vi "NT Write Generic Value.vi"(8 "error in":errorcluster, 9 "Owning Write":bool, 10 "Field Value":T1, 11 "Name":string="Boolean") -> (0 "error out":errorcluster)   [LabVIEW 2017]
doc: "Write the generic cluster data for a variable into the named entry."
uses:
  <vilib>/Rock Robotics/Network Tables/Field Data.ctl
  <vilib>/Rock Robotics/Network Tables/Field Type.ctl
  <vilib>/Rock Robotics/Network Tables/Sequence.ctl
  <vilib>/Rock Robotics/Network Tables/Make Table Operation.ctl
  <vilib>/Rock Robotics/Network Tables/Manage Dirty Field ID List.vi
  <vilib>/Rock Robotics/Network Tables/NT Globals.vi
  <vilib>/Rock Robotics/Network Tables/Update Other Clients.vi
  <vilib>/Rock Robotics/Network Tables/Build Entry Assign Buffer.vi
  <vilib>/Rock Robotics/Network Tables/Field Data Manager.vi
  <vilib>/Rock Robotics/Network Tables/Usage Statistics.vi
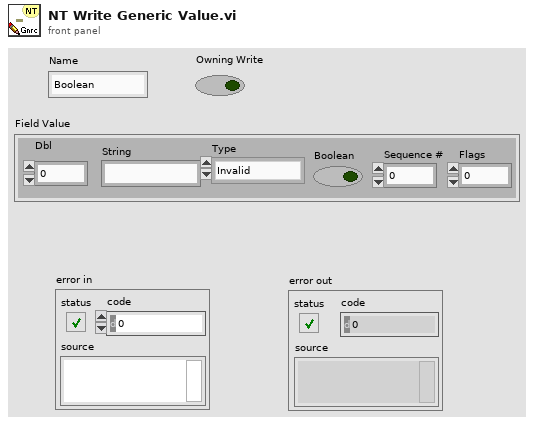
[diagram p1: front panel]
types:
  T1 = typedef "Field Data.ctl" = cluster{"Dbl":dbl, "String":string, "Type":T2, "Boolean":bool, "Sequence #":T3, "Flags":u8}
  T2 = typedef "Field Type.ctl" = enum8{"Invalid", "Bool", "Numeric", "String", "Raw", "Boolean Array", "Numeric Array", "String Array", "RPC"}
  T3 = typedef "Sequence.ctl" = u16
  T4 = typedef "Make Table Operation.ctl" = enum16{"Get or Add Field", "Get Field or Add Temp", "Replace Temp ID", "Get Field ID - No Add", "Get Table Field IDs", "Get Field ID Info", "Move Field to Temp", "Validate", "Remove Field", "Remove All"}
  T5 = typedef "Field ID.ctl" = i32
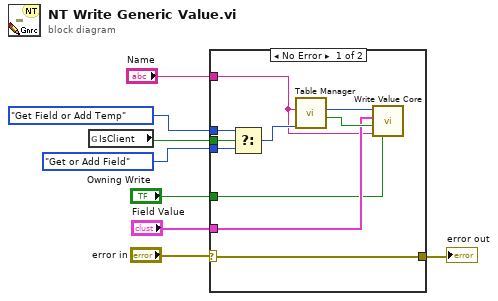
[diagram p0: block diagram]
diagram:
  n1 = global read "NT Globals.vi" "IsClient"() -> (w7:bool)
  n2 = case shown="No Error" "error in" {
    selector: "error in" -> [w11 w19]
    tunnel: "Name" -> [w10 _]
    tunnel: w7 -> [w17 _]
    tunnel: Make_Table_Operation."Get or Add Field" ("Operation") -> [w16 _]
    tunnel: Make_Table_Operation."Get Field or Add Temp" ("Operation") -> [w15 _]
    tunnel: "Field Value" -> [w12 _]
    tunnel: [w11 w19] -> w2
    tunnel: "Owning Write" -> [w9 _]
    frame No Error {
      n3 = Select(t=w15, s=w17, f=w16) -> (s? t:f=w14:T4)
      n4 = call <vilib>:"Table Manager.vi"("Operation"=w14, "Entry Name"=w10) -> ("Success"=w18:bool, "Entry ID"=w13:T5)  [unwired: 6 in, 2 out]
      n5 = call <vilib>:"Write Value Core.vi"("Owning Write"=w9, "Name"=w10, "Existing"=w18, "Field Value"=w12, "Field ID"=w13) -> ()  [unwired: 6 in, 1 out]
    }
    frame Error {
    }
  }
  "error out" <- w2
